vi "Datasheet Find PIM Up Dn Max.vi"(9 "im power waveform":dbl[](array[numeric]), 10 "tx1 frequency":dbl[](array[numeric]), 11 "direction":string) -> (2 "max":dbl, 3 "max index":i32)   [LabVIEW 2011]
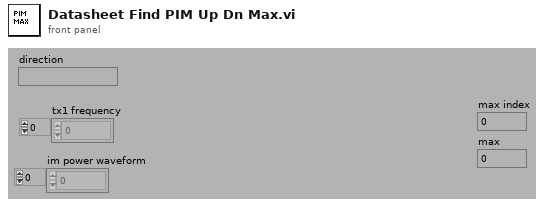
[diagram p1: front panel]
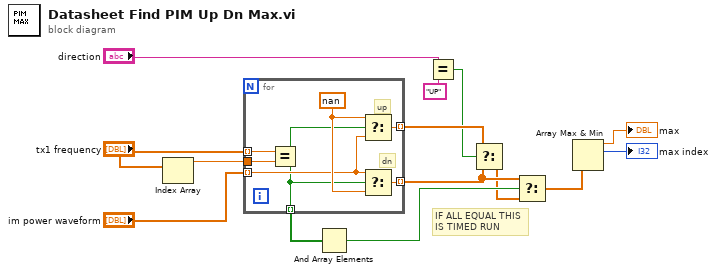
[diagram p0: block diagram]
diagram:
  # "IF ALL EQUAL THIS\nIS TIMED RUN"
  n1 = Index Array(array="tx1 frequency") -> (element=w8:dbl)  [unwired: 1 in]
  n2 = for {
    tunnel: "tx1 frequency" -> [w21] mode=indexing
    tunnel: w8 -> [w20]
    tunnel: "im power waveform" -> [w17] mode=indexing
    tunnel: [w19] -> w4 mode=indexing
    tunnel: [w16] -> w12 mode=indexing
    tunnel: [w15] -> w5 mode=indexing
    w18 = nan ("y")
    # "dn"
    # "up"
    n3 = Equal?(x=w21, y=w20) -> (x = y?=w15:bool)
    n4 = Select(t=w18, s=w15, f=w17) -> (s? t:f=w16:dbl)
    n5 = Select(t=w17, s=w15, f=w18) -> (s? t:f=w19:dbl)
  }
  n6 = And Array Elements(Boolean array=w5) -> (logical AND=w3:bool)
  n7 = Equal?(x="direction", y="UP") -> (x = y?=w6:bool)
  n8 = Select(t=w12, s=w6, f=w4) -> (s? t:f=w2:dbl[])
  n9 = Select(t=w4, s=w3, f=w2) -> (s? t:f=w1:dbl[])
  n10 = Array Max & Min(array=w1) -> (max value=→"max":dbl, max index (indices)=→"max index":i32)  [unwired: 2 out]
